vi "find steer angle errors.vi"(10 "Desired Motion":T1, 11 "Actual Angles":T1) -> (3 "Commanded Motion":T1)   [LabVIEW 2019]
uses:
  Controls/Robot Pivot Motion Commands.ctl
  Controls/Pivot Motor Commands.ctl
  Controls/Robot Drive Mode.ctl
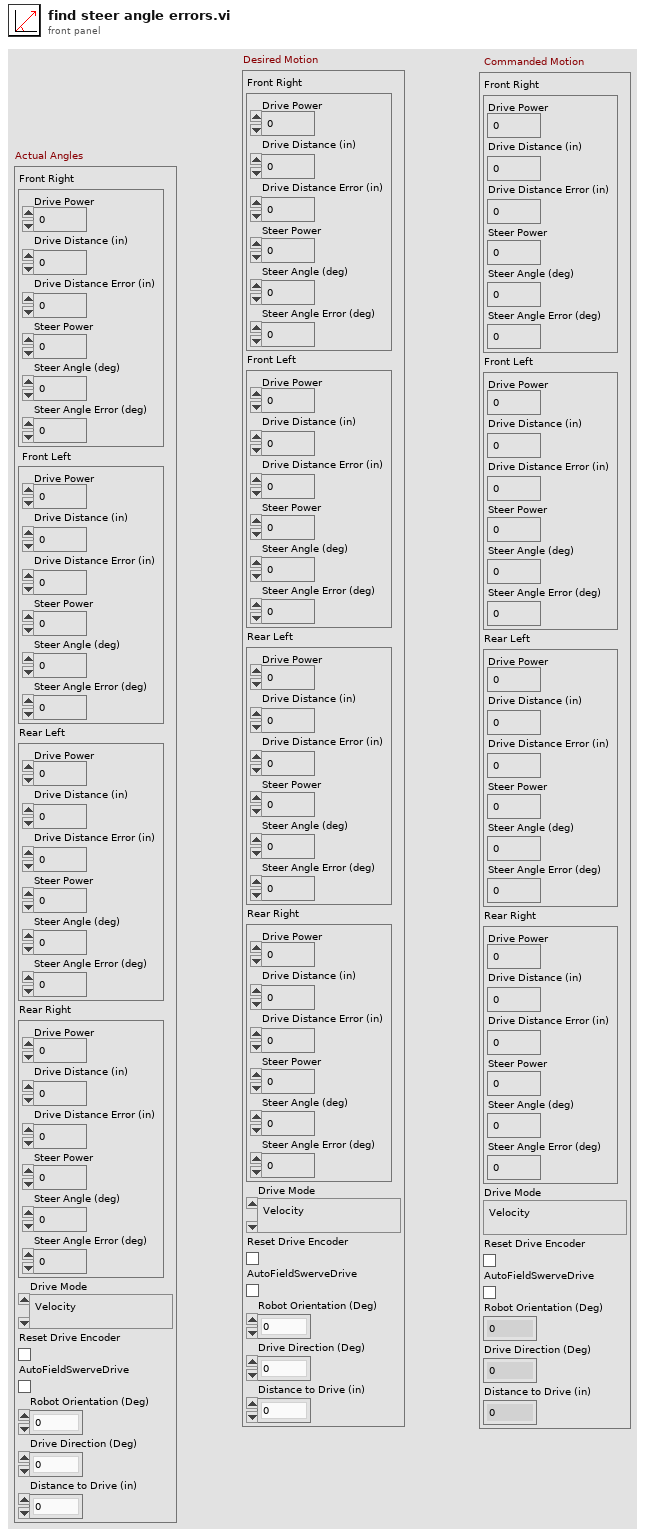
[diagram p1: front panel]
types:
  T1 = typedef "Robot Pivot Motion Commands.ctl" = cluster{"Front Right":T2, "Front Left":T2, "Rear Left":T2, "Rear Right":T2, "Drive Mode":T3, "Reset Drive Encoder":bool, "AutoFieldSwerveDrive":bool, "Robot Orientation (Deg)":dbl, "Drive Direction (Deg)":dbl, "Distance to Drive (in)":dbl}
  T2 = typedef "Pivot Motor Commands.ctl" = cluster{"Drive Power":dbl, "Drive Distance (in)":dbl, "Drive Distance Error (in)":dbl, "Steer Power":dbl, "Steer Angle (deg)":dbl, "Steer Angle Error (deg)":dbl}
  T3 = typedef "Robot Drive Mode.ctl" = enum16{"Velocity", "Distance"}
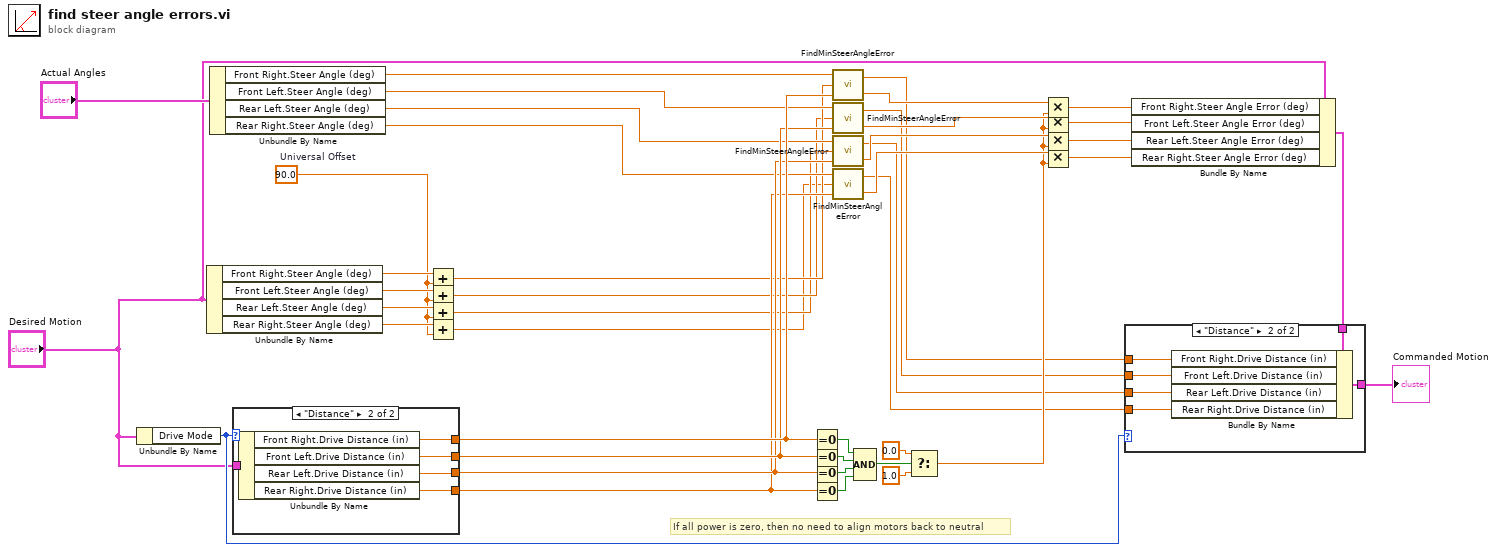
[diagram p0: block diagram]
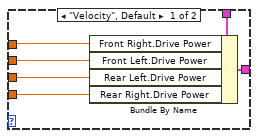
[diagram p2: hidden frame]
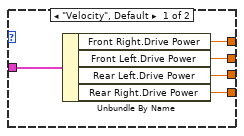
[diagram p3: hidden frame]
diagram:
  w21 = 90.0  # Universal Offset
  # "If all power is zero, then no need to align motors back to neutral"
  n1 = Unbundle By Name("Desired Motion") -> ("Drive Mode"=w16:T3)
  n2 = Unbundle By Name("Desired Motion") -> ("Front Right.Steer Angle (deg)"=w25:dbl, "Front Left.Steer Angle (deg)"=w24:dbl, "Rear Left.Steer Angle (deg)"=w23:dbl, "Rear Right.Steer Angle (deg)"=w22:dbl)
  n3 = Unbundle By Name("Actual Angles") -> ("Front Right.Steer Angle (deg)"=w8:dbl, "Front Left.Steer Angle (deg)"=w7:dbl, "Rear Left.Steer Angle (deg)"=w6:dbl, "Rear Right.Steer Angle (deg)"=w5:dbl)
  n4 = case shown="\"Distance\"" w16 {
    tunnel: "Desired Motion" -> [w47 w52]
    tunnel: [w46 w51] -> w20
    tunnel: [w45 w50] -> w19
    tunnel: [w44 w49] -> w18
    tunnel: [w43 w48] -> w17
    frame "Velocity", Default {
      n5 = Unbundle By Name(w47) -> ("Front Right.Drive Power"=w46:dbl, "Front Left.Drive Power"=w45:dbl, "Rear Left.Drive Power"=w44:dbl, "Rear Right.Drive Power"=w43:dbl)
    }
    frame "Distance" {
      n6 = Unbundle By Name(w52) -> ("Front Right.Drive Distance (in)"=w51:dbl, "Front Left.Drive Distance (in)"=w50:dbl, "Rear Left.Drive Distance (in)"=w49:dbl, "Rear Right.Drive Distance (in)"=w48:dbl)
    }
  }
  n7 = Add(x=w25, y=w21) -> (x+y=w4:dbl)
  n8 = Add(x=w24, y=w21) -> (x+y=w3:dbl)
  n9 = Add(x=w23, y=w21) -> (x+y=w2:dbl)
  n10 = Add(x=w22, y=w21) -> (x+y=w1:dbl)
  n11 = Equal To 0?(x=w20) -> (x = 0?=w34:bool)
  n12 = Equal To 0?(x=w19) -> (x = 0?=w33:bool)
  n13 = Equal To 0?(x=w18) -> (x = 0?=w32:bool)
  n14 = Equal To 0?(x=w17) -> (x = 0?=w31:bool)
  n15 = call "FindMinSteerAngleError.vi"("Motor Power"=w20, "Desired Angle"=w4, "Actual Angle"=w8) -> ("Angle Error"=w42:dbl, "Motor Power"=w15:dbl)
  n16 = call "FindMinSteerAngleError.vi"("Motor Power"=w19, "Desired Angle"=w3, "Actual Angle"=w7) -> ("Angle Error"=w41:dbl, "Motor Power"=w14:dbl)
  n17 = call "FindMinSteerAngleError.vi"("Motor Power"=w18, "Desired Angle"=w2, "Actual Angle"=w6) -> ("Angle Error"=w40:dbl, "Motor Power"=w13:dbl)
  n18 = call "FindMinSteerAngleError.vi"("Motor Power"=w17, "Desired Angle"=w1, "Actual Angle"=w5) -> ("Angle Error"=w39:dbl, "Motor Power"=w12:dbl)
  n19 = Compound Arithmetic op=AND(w34, w33, w32, w31) -> (w30:bool)
  n20 = Select(t=0.0, s=w30, f=1.0) -> (s? t:f=w27:dbl)
  n21 = Multiply(x=w42, y=w27) -> (x*y=w38:dbl)
  n22 = Multiply(x=w41, y=w27) -> (x*y=w37:dbl)
  n23 = Multiply(x=w40, y=w27) -> (x*y=w36:dbl)
  n24 = Multiply(x=w39, y=w27) -> (x*y=w35:dbl)
  n25 = Bundle By Name(cluster="Desired Motion", "Front Right.Steer Angle Error (deg)"=w38, "Front Left.Steer Angle Error (deg)"=w37, "Rear Left.Steer Angle Error (deg)"=w36, "Rear Right.Steer Angle Error (deg)"=w35) -> (w26:T1)
  n26 = case shown="\"Distance\"" w16 {
    tunnel: w26 -> [w58 w64]
    tunnel: [w57 w59] -> w9
    tunnel: w15 -> [w56 w63]
    tunnel: w14 -> [w55 w62]
    tunnel: w13 -> [w54 w61]
    tunnel: w12 -> [w53 w60]
    frame "Velocity", Default {
      n27 = Bundle By Name(cluster=w58, "Front Right.Drive Power"=w56, "Front Left.Drive Power"=w55, "Rear Left.Drive Power"=w54, "Rear Right.Drive Power"=w53) -> (w57:T1)
    }
    frame "Distance" {
      n28 = Bundle By Name(cluster=w64, "Front Right.Drive Distance (in)"=w63, "Front Left.Drive Distance (in)"=w62, "Rear Left.Drive Distance (in)"=w61, "Rear Right.Drive Distance (in)"=w60) -> (w59:T1)
    }
  }
  "Commanded Motion" <- w9
